vi "FPGA_EncoderWriteConfiguration.vi"(4 "IndexActiveHigh":bool=TRUE, 5 "IndexSource":T1={"DevStatus"={"status"=FALSE, "code"=0, "source"=""}, "AnalogTriggerMode?"=FALSE, "DigitalMode"={"DIO Channel"=enum."DIO 1"}, "AnalogTriggerMode"={"AnalogTriggerIndex"=enum."Trig 0", "OutputType"=enum."InWindow"}}, 6 "Reverse?":bool, 7 "Enable":bool, 8 "error in (no error)":errorcluster, 9 "BSource":T1={"DevStatus"={"status"=FALSE, "code"=0, "source"=""}, "AnalogTriggerMode?"=FALSE, "DigitalMode"={"DIO Channel"=enum."DIO 1"}, "AnalogTriggerMode"={"AnalogTriggerIndex"=enum."Trig 0", "OutputType"=enum."InWindow"}}, 10 "ASource":T1={"DevStatus"={"status"=FALSE, "code"=0, "source"=""}, "AnalogTriggerMode?"=FALSE, "DigitalMode"={"DIO Channel"=enum."DIO 1"}, "AnalogTriggerMode"={"AnalogTriggerIndex"=enum."Trig 0", "OutputType"=enum."InWindow"}}, 11 "EncoderDevRef":T5) -> (0 "error out":errorcluster, 3 "EncoderDevRef":T5)   [LabVIEW 2017]
uses:
  <vilib>/Rock Robotics/SystemInterfaces/Encoder/FPGA_EncoderDevRef.ctl
  <vilib>/Rock Robotics/SystemInterfaces/Encoder/FPGA_EncoderIdx.ctl
  <vilib>/Rock Robotics/SystemInterfaces/CounterEncoderSourceConvertion/FPGA_CounterEncoderSourceConvertionLVSourceType.ctl
  <vilib>/Rock Robotics/SystemInterfaces/DIO/FPGA_DIODigitalSourceChannel.ctl
  <vilib>/Rock Robotics/SystemInterfaces/AnalogTrigger/FPGA_AnalogTriggerIndex.ctl
  <vilib>/Rock Robotics/SystemInterfaces/AnalogTrigger/FPGA_AnalogTriggerOutType.ctl
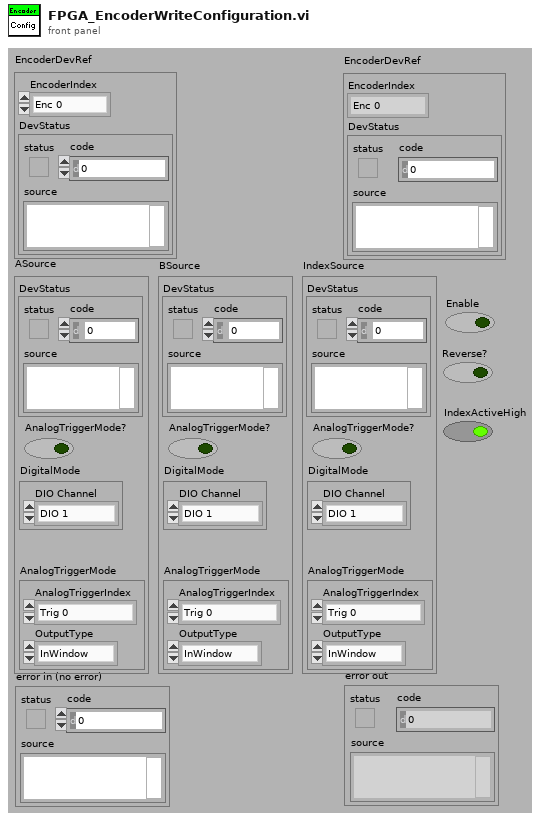
[diagram p1: front panel]
types:
  T1 = typedef "FPGA_CounterEncoderSourceConvertionLVSourceType.ctl" = cluster{"DevStatus":errorcluster, "AnalogTriggerMode?":bool, "DigitalMode":cluster{"DIO Channel":T2}, "AnalogTriggerMode":cluster{"AnalogTriggerIndex":T3, "OutputType":T4}}
  T2 = typedef "FPGA_DIODigitalSourceChannel.ctl" = enum8{"DIO 0", "DIO 1", "DIO 2", "DIO 3", "DIO 4", "DIO 5", "DIO 6", "DIO 7", "DIO 8", "DIO 9", "DIO MXP 0", "DIO MXP 1", "DIO MXP 2", "DIO MXP 3", "DIO MXP 4", "DIO MXP 5", "DIO MXP 6", "DIO MXP 7", "DIO MXP 8", "DIO MXP 9", "DIO MXP 10", "DIO MXP 11", "DIO MXP 12", "DIO MXP 13", "DIO MXP 14", "DIO MXP 15", "Disabled"}
  T3 = typedef "FPGA_AnalogTriggerIndex.ctl" = enum8{"Trig 0", "Trig 1", "Trig 2", "Trig 3", "Trig 4", "Trig 5", "Trig 6", "Trig 7", "Invalid"}
  T4 = typedef "FPGA_AnalogTriggerOutType.ctl" = enum16{"InWindow", "TriggerState", "Rising", "Falling"}
  T5 = typedef "FPGA_EncoderDevRef.ctl" = cluster{"EncoderIndex":T6, "DevStatus":errorcluster}
  T6 = typedef "FPGA_EncoderIdx.ctl" = enum8{"Enc 0", "Enc 1", "Enc 2", "Enc 3", "Enc 4", "Enc 5", "Enc 6", "Enc 7", "Invalid"}
  T7 = cluster{"ASource":cluster{"Channel":fxp<+,4,4>, "Module":fxp<+,1,1>, "AnalogTrigger":bool}, "BSource":cluster{"Channel":fxp<+,4,4>, "Module":fxp<+,1,1>, "AnalogTrigger":bool}, "IndexSource":cluster{"Channel":fxp<+,4,4>, "Module":fxp<+,1,1>, "AnalogTrigger":bool}, "IndexActiveHigh":bool, "Reverse":bool, "Enable":bool}
  T8 = cluster{"Channel":fxp<+,4,4>, "Module":fxp<+,1,1>, "AnalogTrigger":bool}
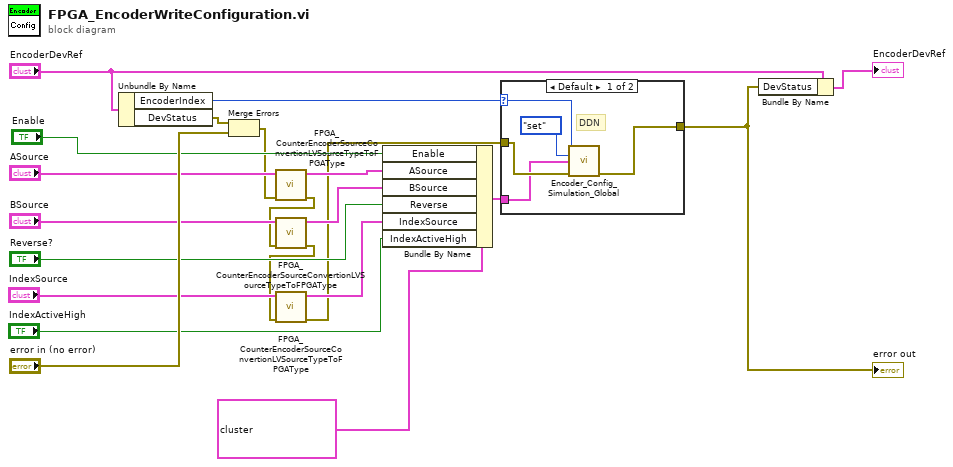
[diagram p0: block diagram]
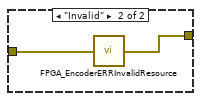
[diagram p2: hidden frame]
diagram:
  n1 = Unbundle By Name("EncoderDevRef") -> ("EncoderIndex"=w10:T6, "DevStatus"=w3:errorcluster)
  n2 = Merge Errors(w3, "error in (no error)") -> (w2:errorcluster)
  n3 = call <vilib>:"FPGA_CounterEncoderSourceConvertionLVSourceTypeToFPGAType.vi"("error in (no error)"=w2, "DigitalSource"="ASource") -> ("error out"=w6:errorcluster, "FPGASource"=w9:T8)  [unwired: 8 out]
  n4 = call <vilib>:"FPGA_CounterEncoderSourceConvertionLVSourceTypeToFPGAType.vi"("error in (no error)"=w6, "DigitalSource"="BSource") -> ("error out"=w5:errorcluster, "FPGASource"=w8:T8)  [unwired: 8 out]
  n5 = call <vilib>:"FPGA_CounterEncoderSourceConvertionLVSourceTypeToFPGAType.vi"("error in (no error)"=w5, "DigitalSource"="IndexSource") -> ("error out"=w4:errorcluster, "FPGASource"=w7:T8)  [unwired: 8 out]
  n6 = Bundle By Name(cluster=T7 {"ASource"={"Channel"=0.0, "Module"=0.0, "AnalogTrigger"=FALSE}, "BSource"={"Channel"=0.0, "Module"=0.0, "AnalogTrigger"=FALSE}, "IndexSource"={"Channel"=0.0, "Module"=0.0, "AnalogTrigger"=FALSE}, "IndexActiveHigh"=TRUE, "Reverse"=FALSE, "Enable"=FALSE} ("Encoder0.Config"), "Enable"="Enable", "ASource"=w9, "BSource"=w8, "Reverse"="Reverse?", "IndexSource"=w7, "IndexActiveHigh"="IndexActiveHigh") -> (w1:T7)
  n7 = case shown="Default" w10 {
    selector: w10 -> [w23 _]
    tunnel: [w26 w27] -> w18
    tunnel: w1 -> [w24 _]
    tunnel: w4 -> [w25 w28]
    frame Default {
      # "DDN"
      n8 = call <vilib>:"Encoder_Config_Simulation_Global.vi"("EncoderIndex"=w23, "menu"=enum16{"set", "get", "delete"}."set", "Encoder Config set"=w24, "error in (no error)"=w25) -> ("error out"=w26:errorcluster)  [unwired: 10 in, 1 out]
    }
    frame "Invalid" {
      n9 = call <vilib>:"FPGA_EncoderERRInvalidResource.vi"("error in (no error)"=w28) -> ("error out"=w27:errorcluster)
    }
  }
  "error out" <- w18
  n10 = Bundle By Name(cluster="EncoderDevRef", "DevStatus"=w18) -> (→"EncoderDevRef":T5)
